vi "Write Available Data Names.vi"(6 "Available Data Names":string[](array[string]), 11 "Handle Drop Msg in":refnum<class "Handle Drop Msg.lvclass">) -> (3 "Handle Drop Msg out":refnum<class "Handle Drop Msg.lvclass">)   [LabVIEW 2017, in "Handle Drop Msg.lvclass"]
uses:
  <vilib>/gpm_packages/@cs/Test-executive-builder/Source/Test Executive Builder View/Test Executive Builder View Messages/Handle Drop Msg/Handle Drop Msg.lvclass
  <vilib>/gpm_packages/@cs/Test-executive-builder/Source/Test Executive Builder View/Test Executive Builder View Messages/Handle Drop Msg/Handle Drop Msg.lvclass/Handle Drop Msg.ctl
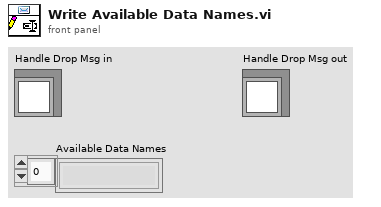
[diagram p1: front panel]
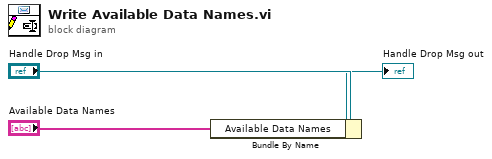
[diagram p0: block diagram]
diagram:
  n1 = Bundle By Name(cluster="Handle Drop Msg in", "Available Data Names"="Available Data Names") -> (→"Handle Drop Msg out":refnum<class "Handle Drop Msg.lvclass">)
